vi "thermo_open.vi"(7 "force open":bool, 8 "error in":errorcluster, 11 "thermo in":T1={"type"=enum."COMET Tx5xx (ethernet)", "comment"="", "tag"="", "refresh"=0.0, "IP"="", "port"=0, "VISA"="", "last readout"=timestamp(0 s since 1904-01-01), "TCP ref"=refnum, "VISA sess"="", "idn"="", "press"=0.0, "RH"=0.0, "temp"=0.0, "pres cor"=[], "RH cor"=[], "temp cor"=[], "try left"=0, "failed"=FALSE, "RTD set"=[], "RTD inv"=[], "range"=0.0, "net mode"=enum."MODBUS", "try fail"=enum."Stop trying - return NaN", "timeout [s]"=0.0, "max retries"=0, "sim t [deg]"=0.0} {"RTD inv" format="%.1f"; "RTD set" format="%.1f"; "temp cor" format="%.1f"; "RH cor" format="%.1f"; "pres cor" format="%.1f"; "refresh" min=0.1 max=1000.0 format="%.2f"}) -> (0 "error out":errorcluster, 1 "instrument name":string, 2 "ID string":string, 3 "thermo out":T1={"type"=enum."COMET Tx5xx (ethernet)", "comment"="", "tag"="", "refresh"=0.0, "IP"="", "port"=0, "VISA"="", "last readout"=timestamp(0 s since 1904-01-01), "TCP ref"=refnum, "VISA sess"="", "idn"="", "press"=0.0, "RH"=0.0, "temp"=0.0, "pres cor"=[], "RH cor"=[], "temp cor"=[], "try left"=0, "failed"=FALSE, "RTD set"=[], "RTD inv"=[], "range"=0.0, "net mode"=enum."MODBUS", "try fail"=enum."Stop trying - return NaN", "timeout [s]"=0.0, "max retries"=0, "sim t [deg]"=0.0} {"RTD inv" format="%.1f"; "RTD set" format="%.1f"; "temp cor" format="%.1f"; "RH cor" format="%.1f"; "pres cor" format="%.1f"; "refresh" min=0.1 max=1000.0 format="%.2f"})   [LabVIEW 2020]
uses:
  thermo.ctl
  thermo_types.ctl
  Thermometer Fail Action.ctl
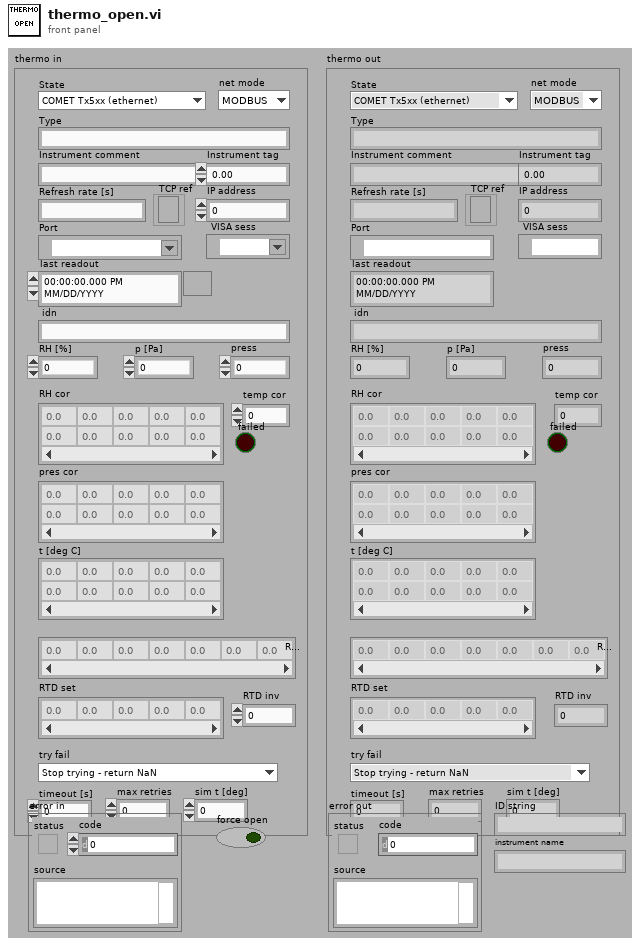
[diagram p1: front panel]
types:
  T1 = typedef "thermo.ctl" = cluster{"type":T2, "comment":string, "tag":string, "refresh":dbl, "IP":string, "port":u16, "VISA":refnum<visa-resource-name>, "last readout":timestamp, "TCP ref":refnum<k5>, "VISA sess":refnum<visa-resource-name>, "idn":string, "press":dbl, "RH":dbl, "temp":dbl, "pres cor":dbl[][], "RH cor":dbl[][], "temp cor":dbl[][], "try left":i32, "failed":bool, "RTD set":dbl[], "RTD inv":dbl[], "range":dbl, "net mode":enum16{"MODBUS", "HTTP"}, "try fail":T3, "timeout [s]":dbl, "max retries":i32, "sim t [deg]":dbl}
  T2 = typedef "thermo_types.ctl" = enum16{"Disabled", "Simulated", "COMET Tx5xx (ethernet)", "Keithley 2002 (GPIB) + RTD", "Agilent 344xx (GPIB) + RTD"}
  T3 = typedef "Thermometer Fail Action.ctl" = enum16{"Stop trying - keep last value", "Stop trying - return NaN", "Generate error - stop sweep"}
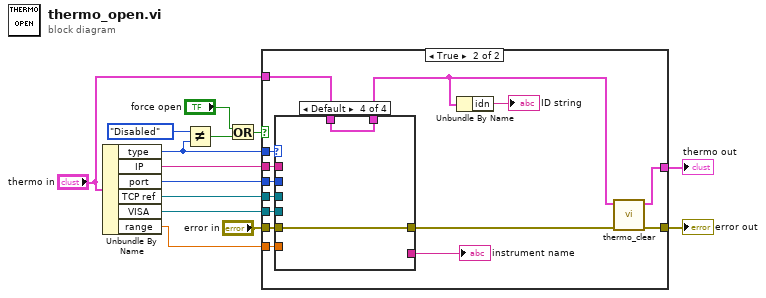
[diagram p0: block diagram]
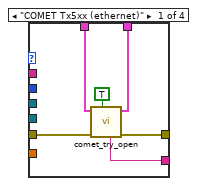
[diagram p3: hidden frame]
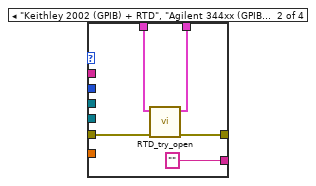
[diagram p4: hidden frame]
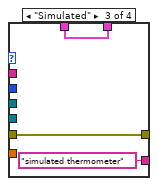
[diagram p5: hidden frame]
diagram:
  n1 = Unbundle By Name("thermo in") -> ("type"=w3:T2, "IP"=w12:string, "port"=w11:u16, "TCP ref"=w7:refnum<k5>, "VISA"=w5:refnum<visa-resource-name>, "range"=w4:dbl)
  n2 = Not Equal?(x=thermo_types."Disabled", y=w3) -> (x != y?=w2:bool)
  n3 = Or(x="force open", y=w2) -> (x .or. y?=w13:bool)
  n4 = case shown="True" w13 {
    tunnel: w3 -> [_ w30]
    tunnel: w12 -> [_ w29]
    tunnel: w11 -> [_ w28]
    tunnel: "thermo in" -> [w15 w20]
    tunnel: "error in" -> [w16 w27]
    tunnel: [w16 w24] -> w9
    tunnel: w7 -> [_ w26]
    tunnel: [w15 w22] -> w6
    tunnel: w5 -> [_ w21]
    tunnel: w4 -> [_ w19]
    frame False {
    }
    frame True {
      n5 = case shown="Default" w30 {
        tunnel: w29 -> [_ _ _ _]
        tunnel: w28 -> [_ _ _ _]
        tunnel: w27 -> [w36 w40 w44 w45]
        tunnel: [w35 w39 w44 w45] -> w23
        tunnel: w26 -> [_ _ _ _]
        tunnel: [w32 "" ("name") "simulated thermometer" ("name") _] -> w25
        tunnel: w21 -> [_ _ _ _]
        tunnel: w20 -> [w34 w37 w42 w46]
        tunnel: [w33 w38 w42 w46] -> w18
        tunnel: w19 -> [_ _ _ _]
        frame "COMET Tx5xx (ethernet)" {
          n6 = call "comet_try_open.vi"("idn"=TRUE, "error in"=w36, "thermo in"=w34) -> ("error out"=w35:errorcluster, "thermo cluster"=w33:T1, "name"=w32:string)  [unwired: 6 in]
        }
        frame "Keithley 2002 (GPIB) + RTD", "Agilent 344xx (GPIB) + RTD" {
          n7 = call "RTD_try_open.vi"("error in"=w40, "thermo in"=w37) -> ("error out"=w39:errorcluster, "thermo out"=w38:T1)  [unwired: 8 in]
        }
        frame "Simulated" {
        }
        frame Default {
        }
      }
      "instrument name" <- w25
      n8 = Unbundle By Name(w18) -> ("idn"=→"ID string":string)
      n9 = call "thermo_clear.vi"("error in (no error)"=w23, "thermo in"=w18) -> ("error out"=w24:errorcluster, "thermo out"=w22:T1)  [unwired: 8 in]
    }
  }
  "error out" <- w9
  "thermo out" <- w6
